vi "创建路径.vi"(8 "error in (no error)":errorcluster caption="错误输入（无错误）", 11 "path":path caption="路径") -> (0 "error out":errorcluster caption="错误输出", 3 "path out":path)   [LabVIEW 2020]
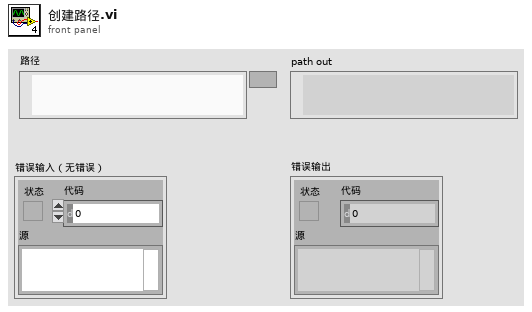
[diagram p1: front panel]
types:
  T1 = enum16{"open", "replace", "create", "open or create", "replace or create", "replace or create with confirmation"}
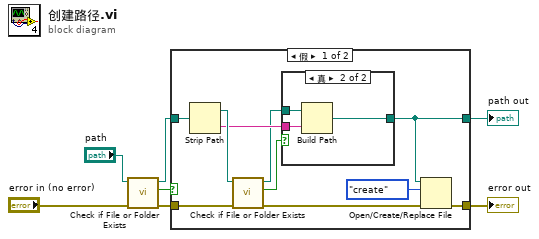
[diagram p0: block diagram]
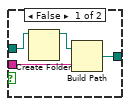
[diagram p2: hidden frame]
diagram:
  n1 = call <vilib>:"Check if File or Folder Exists.vi"("error in (no error)"="error in (no error)", "path"="path") -> ("error out"=w4:errorcluster, "file or folder exists?"=w7:bool, "dup path"=w6:path)  [unwired: 7 in]
  n2 = case shown="假" w7 {
    tunnel: w6 -> [w16 w26]
    tunnel: [w11 w26] -> w1
    tunnel: w4 -> [w10 w25]
    tunnel: [w8 w25] -> w3
    frame False {
      n3 = Strip Path(path=w16) -> (stripped path=w15:path, name=w13:string)
      n4 = call <vilib>:"Check if File or Folder Exists.vi"("error in (no error)"=w10, "path"=w15) -> ("error out"=w9:errorcluster, "file or folder exists?"=w14:bool, "dup path"=w12:path)  [unwired: 7 in]
      n5 = case shown="真" w14 {
        tunnel: w13 -> [w19 w23]
        tunnel: w12 -> [w21 w24]
        tunnel: [w18 w22] -> w11
        frame False {
          n6 = Create Folder(path (use dialog)=w21) -> (created path=w20:path)  [unwired: 2 in, 2 out]
          n7 = Build Path(base path=w20, name or relative path=w19) -> (appended path=w18:path)
        }
        frame True {
          n8 = Build Path(base path=w24, name or relative path=w23) -> (appended path=w22:path)
        }
      }
      n9 = Open/Create/Replace File(file path (use dialog)=w11, error in=w9, operation (0:open)=T1."create" ("操作(0:open)")) -> (error out=w8:errorcluster)  [unwired: 3 in, 2 out]
    }
    frame True {
    }
  }
  "error out" <- w3
  "path out" <- w1
